vi "LVProjectShortcut_RunView.vi"(8 "error in (no error)":errorcluster, 11 "Object":T1) -> (0 "error out":errorcluster)   [LabVIEW 2017]
doc: "Calls the View VI."
uses:
  <resource>/Framework/Providers/API/ItemRef.ctl
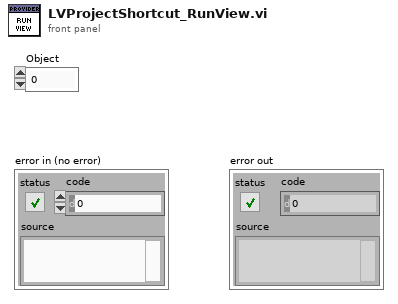
[diagram p1: front panel]
types:
  T1 = typedef "ItemRef.ctl" = u64
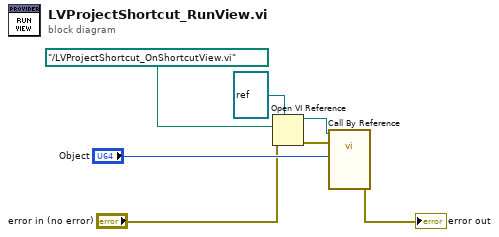
[diagram p0: block diagram]
diagram:
  n1 = Open VI Reference(type specifier VI Refnum (for type only)=refnum<vi> refnum, vi path=path "../LVProjectShortcut_OnShortcutView.vi", error in (no error)="error in (no error)") -> (vi reference=w2:refnum<vi>, error out=w1:errorcluster)  [unwired: 3 in]
  n2 = call-by-ref "?"(reference=w2, error in=w1, "Object"="Object") -> (error out=→"error out":errorcluster)  [unwired: 10 in, 2 out]
